vi "RemoveBus.vi"(0 "BusArray":refnum<class "Bus.lvclass">[](array[class]), 1 "BusNumberRef":refnum<vi>, 2 "BusNumber":u8) -> (7 "BusArray":refnum<class "Bus.lvclass">[](array[class]), 8 "BusIndex":i32)   [LabVIEW 2014, in "Visualization.lvlib" / "VisualizeBase_class.lvclass"]
uses:
  VisializeBase_class/VisualizeBase_class.lvclass
  Framework/Bus_class/Bus.lvclass
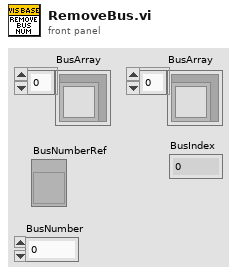
[diagram p1: front panel]
types:
  T1 = typedef "LVStringsAndValuesArrayTypeDef_U8.ctl" = cluster{"String":string, "Value":u8}[]
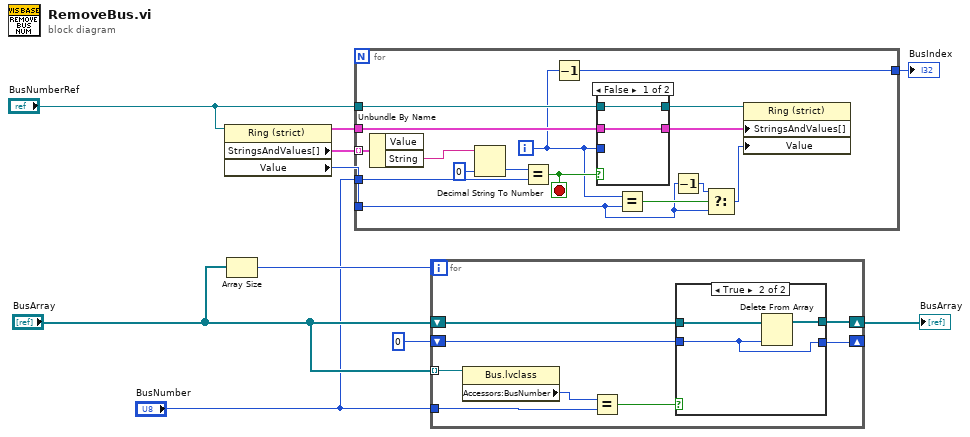
[diagram p0: block diagram]
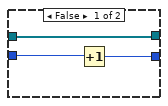
[diagram p2: hidden frame]
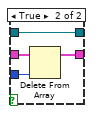
[diagram p3: hidden frame]
diagram:
  n1 = property class="Ring (strict)"(reference="BusNumberRef") -> ("StringsAndValues[]"=w9:T1, "Value"=w8:u8)  [unwired: 1 in, 2 out]
  n2 = Array Size(array="BusArray") -> (size(s)=w4:i32)
  n3 = for {
    tunnel: w9 -> [w25] mode=indexing
    tunnel: "BusNumber" -> [w21]
    tunnel: w9 -> [w20]
    tunnel: w8 -> [w16]
    tunnel: "BusNumberRef" -> [w13]
    tunnel: [w10] -> w6
    i -> [w11]
    stop <- w19 stop-if-true
    n4 = Unbundle By Name(w25) -> ("String"=w24:string)  [unwired: 1 out]
    n5 = Decimal String To Number(string=w24, default (0L)=u8 0 ("default (0 I32)")) -> (number=w22:u8)  [unwired: 1 in, 1 out]
    n6 = Equal?(x=w22, y=w21) -> (x = y?=w19:bool)
    n7 = Decrement(x=w11) -> (x-1=w10:i32)
    n8 = case shown="False" w19 {
      tunnel: w20 -> [w27 w31]
      tunnel: w11 -> [_ w28]
      tunnel: [w27 w30] -> w15
      tunnel: w13 -> [w26 w29]
      tunnel: [w26 w29] -> w12
      frame False {
      }
      frame True {
        n9 = Delete From Array(array=w31, index=w28) -> (array with subset deleted=w30:T1)  [unwired: 1 in, 1 out]
      }
    }
    n10 = Equal?(x=w11, y=w16) -> (x = y?=w18:bool)
    n11 = Decrement(x=w16) -> (x-1=w17:u8)
    n12 = Select(t=w17, s=w18, f=w16) -> (s? t:f=w14:u8)
    n13 = property class="Ring (strict)"(reference=w12, "StringsAndValues[]"=w15, "Value"=w14) -> ()  [unwired: 1 in, 2 out]
  }
  "BusIndex" <- w6
  n14 = for {
    N: w4 -> [_]
    tunnel: "BusNumber" -> [w38]
    shift-right: [w36] -> w5
    shift-left: "BusArray" -> [w35]
    tunnel: "BusArray" -> [w34] mode=indexing
    shift-right: [w32] -> _
    shift-left: 0 -> [w33]
    n15 = property class="Bus.lvclass"(reference=w34) -> ("Accessors:BusNumber"=w39:u8)  [unwired: 1 in, 2 out]
    n16 = Equal?(x=w39, y=w38) -> (x = y?=w37:bool)
    n17 = case shown="True" w37 {
      tunnel: w35 -> [w42 w45]
      tunnel: [w42 w44] -> w36
      tunnel: w33 -> [w41 w43]
      tunnel: [w40 w43] -> w32
      frame False {
        n18 = Increment(x=w41) -> (x+1=w40:i32)
      }
      frame True {
        n19 = Delete From Array(array=w45, index=w43) -> (array with subset deleted=w44:refnum<class "Bus.lvclass">[])  [unwired: 1 in, 1 out]
      }
    }
  }
  "BusArray" <- w5
